vi "calSubset.vi"(4 "offset":i32, 6 "CrsrList":T1, 9 "Decimated 660":dbl[](array[numeric]), 10 "Decimated 532":dbl[](array[numeric]), 11 "GO3 Data":dbl[](array[numeric])) -> (1 "660 Subset":dbl[](array[numeric]), 2 "532 Subset":dbl[](array[numeric]), 3 "Go3 Subset":dbl[](array[numeric]))   [LabVIEW 2011]
uses:
  <vilib>/Utility/miscctls.llb/LVCursorListTypeDef.ctl
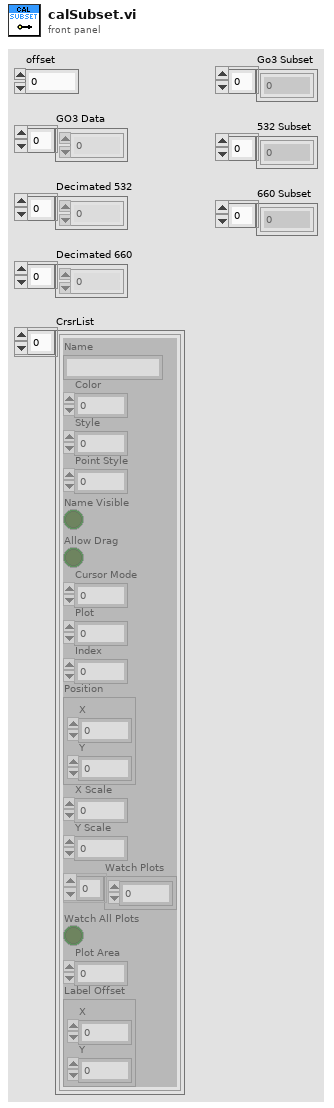
[diagram p1: front panel]
types:
  T1 = typedef "LVCursorListTypeDef.ctl" = cluster{"Name":string, "Color":u32, "Style":u8, "Point Style":u8, "Name Visible":bool, "Allow Drag":bool, "Cursor Mode":u32, "Plot":i32, "Index":i32, "Position":cluster{"X":dbl, "Y":dbl}, "X Scale":u32, "Y Scale":u32, "Watch Plots":i32[], "Watch All Plots":bool, "Plot Area":i32, "Label Offset":cluster{"X":dbl, "Y":dbl}}[]
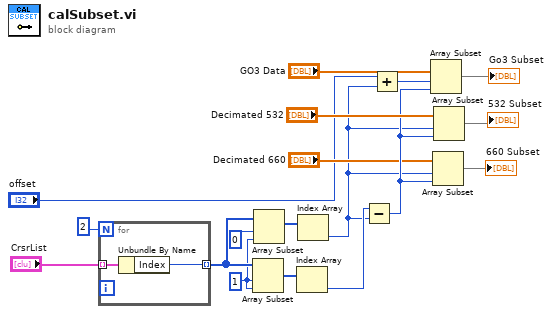
[diagram p0: block diagram]
diagram:
  w4 = 1 ("index")
  n1 = for {
    N: 2 -> [_]
    tunnel: "CrsrList" -> [w20] mode=indexing
    tunnel: [w19] -> w8 mode=indexing
    n2 = Unbundle By Name(w20) -> ("Index"=w19:i32)
  }
  n3 = Array Subset(array=w8, index=w4, length=w4) -> (w10:i32[])
  n4 = Array Subset(array=w8, index=0, length=w4) -> (w9:i32[])
  n5 = Index Array(array=w10) -> (element=w2:i32)  [unwired: 1 in]
  n6 = Index Array(array=w9) -> (element=w1:i32)  [unwired: 1 in]
  n7 = Subtract(x=w2, y=w1) -> (x-y=w16:i32)
  n8 = Add(x="offset", y=w1) -> (x+y=w13:i32)
  n9 = Array Subset(array="GO3 Data", index=w13, length=w16) -> (→"Go3 Subset":dbl[])
  n10 = Array Subset(array="Decimated 660", index=w1, length=w16) -> (→"660 Subset":dbl[])
  n11 = Array Subset(array="Decimated 532", index=w1, length=w16) -> (→"532 Subset":dbl[])
